vi "MEMR-Find Window Length.vi"(0 "State In":T1, 5 "Analysis":T2, 7 "Avg":dbl[][](array[numeric])) -> (8 "Window length":i32)   [LabVIEW 2020]
uses:
  MEMR-Offline Analysis Parameters.ctl
  Typedefs/MEMR-Analysis State.ctl
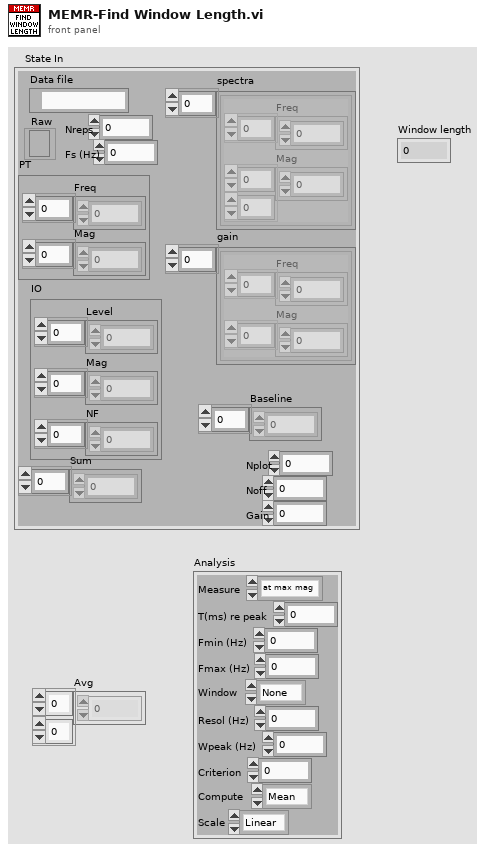
[diagram p1: front panel]
types:
  T1 = typedef "MEMR-Analysis State.ctl" = cluster{"Data file":path, "Raw":refnum<file>, "PT":cluster{"Freq":dbl[], "Mag":dbl[]}, "IO":cluster{"Level":dbl[], "Mag":dbl[], "NF":dbl[]}, "Nreps":i32, "Fs (Hz)":dbl, "Sum":dbl[], "Nplot":i32, "Noff":i32, "Gain":dbl, "spectra":cluster{"Freq":dbl[], "Mag":dbl[][]}[], "gain":cluster{"Freq":dbl[], "Mag":dbl[]}[], "Baseline":dbl[]}
  T2 = typedef "MEMR-Offline Analysis Parameters.ctl" = cluster{"Measure":enum16{"at max mag", "at max gain", "over window", "optimize", "Keefe"}, "T(ms) re peak":dbl, "Fmin (Hz)":dbl, "Fmax (Hz)":dbl, "Window":enum16{"None", "Hanning", "Hamming"}, "Resol (Hz)":dbl, "Wpeak (Hz)":dbl, "Criterion":dbl, "Compute":enum16{"Mean", "Sum"}, "Scale":enum16{"Linear", "Log"}}
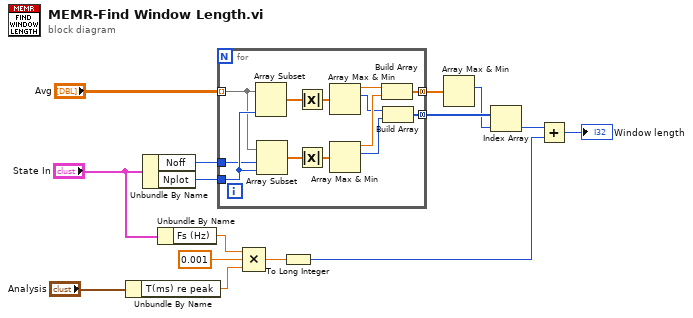
[diagram p0: block diagram]
diagram:
  n1 = Unbundle By Name("Analysis") -> ("T(ms) re peak"=w13:dbl)
  n2 = Unbundle By Name("State In") -> ("Noff"=w9:i32, "Nplot"=w12:i32)
  n3 = Unbundle By Name("State In") -> ("Fs (Hz)"=w6:dbl)
  n4 = for {
    tunnel: w12 -> [w28]
    tunnel: w9 -> [w23]
    tunnel: "Avg" -> [w22] mode=indexing
    tunnel: [w19] -> w4 mode=concatenating
    tunnel: [w16] -> w3 mode=concatenating
    n5 = Array Subset(array=w22, length=w28) -> (w25:dbl[])  [unwired: 1 in]
    n6 = Array Subset(array=w22, index=w23, length=w28) -> (w24:dbl[])
    n7 = Absolute Value(x=w25) -> (abs(x)=w27:dbl[])
    n8 = Absolute Value(x=w24) -> (abs(x)=w26:dbl[])
    n9 = Array Max & Min(array=w27) -> (max value=w21:dbl, max index (indices)=w17:i32)  [unwired: 2 out]
    n10 = Array Max & Min(array=w26) -> (max value=w20:dbl, max index (indices)=w18:i32)  [unwired: 2 out]
    n11 = Build Array(w21, w20) -> (w19:dbl[])
    n12 = Build Array(w17, w18) -> (w16:i32[])
  }
  n13 = Compound Arithmetic op=MULTIPLY(w6, 0.001 ("value"), w13) -> (w15:dbl)
  n14 = To Long Integer(number=w15) -> (32bit integer=w10:i32)
  n15 = Array Max & Min(array=w4) -> (max index (indices)=w2:i32)  [unwired: 3 out]
  n16 = Index Array(array=w3, index=w2) -> (element=w1:i32)
  n17 = Add(x=w1, y=w10) -> (x+y=→"Window length":i32)
